vi "planarFFcircle.vi"(4 "ForceDesired":dbl, 6 "FM--FF":dbl[](array[numeric]), 7 "Radius":dbl, 8 "Center":dbl[](array[numeric]), 9 "ViconData":dbl[](array[numeric])) -> (2 "ActiveFF":bool, 3 "DesiredFM_FF":dbl[](array[numeric]))   [LabVIEW 2017]
uses:
  <vilib>/Analysis/_algsub.llb/Real Vector Norm.vi
  <vilib>/Analysis/NI_AALPro.lvlib
panel:
  out "Current_point":dbl[](array[numeric])
  out "center position":dbl[](array[numeric])
  # "Circle Force Field"
  # "INPUTS"
  # "OUTPUTS:"
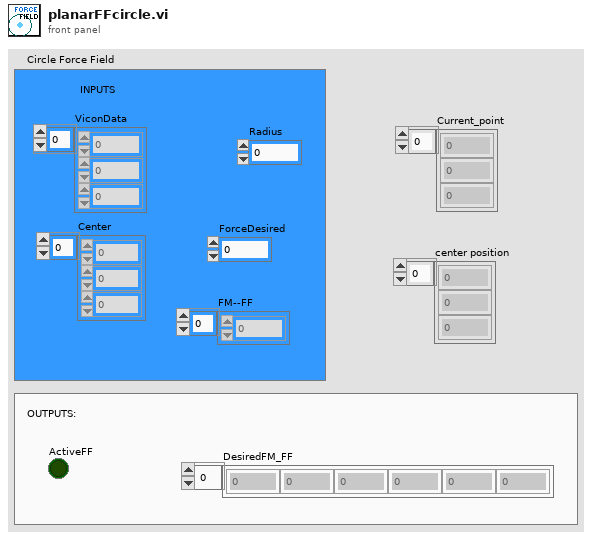
[diagram p1: front panel]
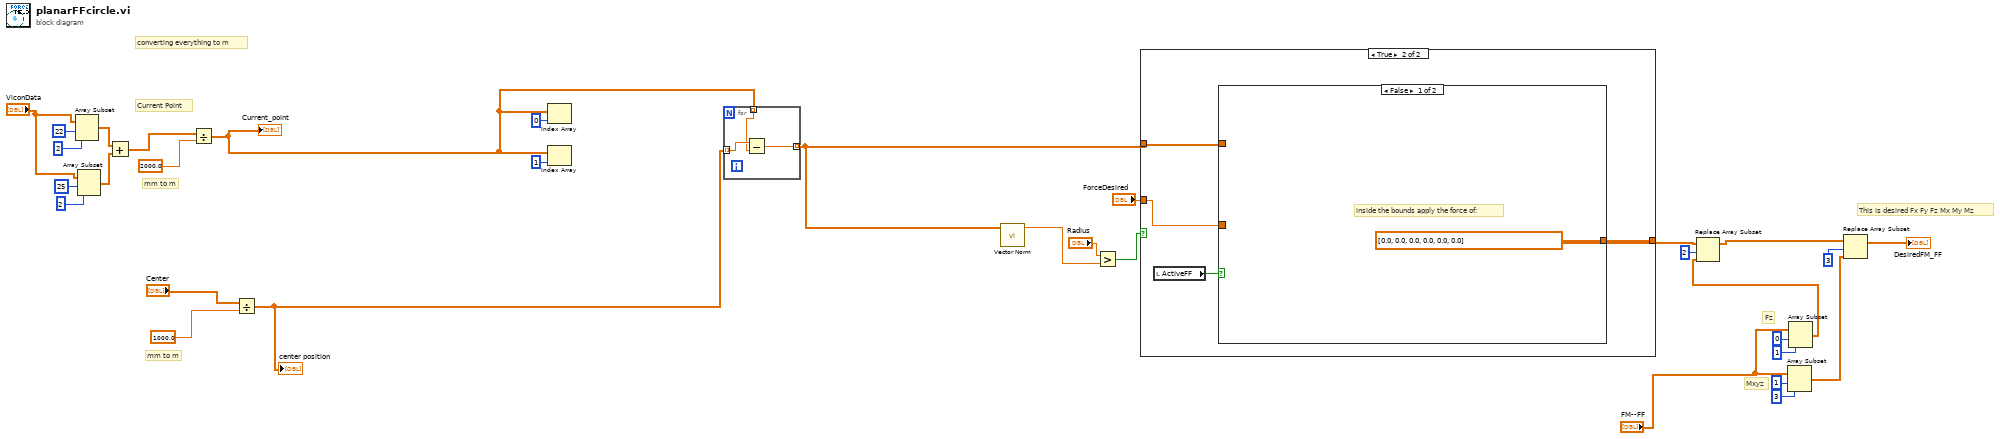
[diagram p0: block diagram]
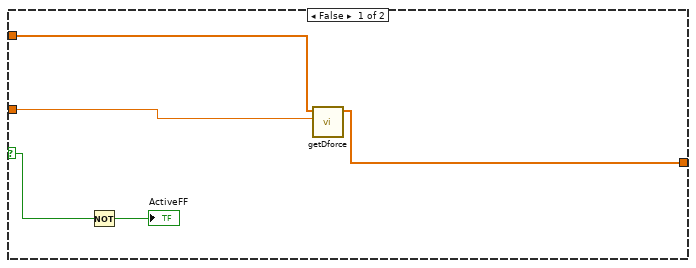
[diagram p2: hidden frame]
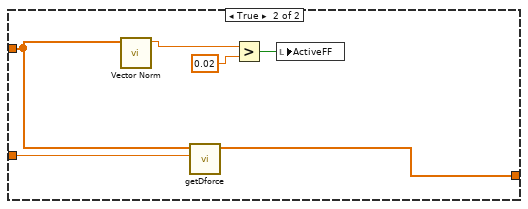
[diagram p3: hidden frame]
diagram:
  # "Current Point"
  # "mm to m"
  # "This is desired Fx Fy Fz Mx My Mz"
  # "converting everything to m"
  # "Fz"
  # "Mxyz"
  # "mm to m"
  n1 = Array Subset(array="ViconData", index=22, length=2) -> (w10:dbl[])
  n2 = Array Subset(array="ViconData", index=25, length=2) -> (w9:dbl[])
  n3 = Add(x=w10, y=w9) -> (x+y=w8:dbl[])
  n4 = Divide(x=w8, y=2000.0) -> (x/y=w7:dbl[])
  "Current_point" <- w7
  n5 = Divide(x="Center", y=1000.0) -> (x/y=w18:dbl[])
  "center position" <- w18
  n6 = Index Array(array=w7, index=0) -> ()  [unwired: 1 out]
  n7 = Index Array(array=w7, index=1) -> ()  [unwired: 1 out]
  n8 = for {
    tunnel: w18 -> [w34] mode=indexing
    tunnel: w7 -> [w33] mode=indexing
    tunnel: [w35] -> w5 mode=indexing
    n9 = Subtract(x=w34, y=w33) -> (x-y=w35:dbl)
  }
  n10 = call-poly <vilib>:"Vector Norm.vi"("Input Vector"=w5) -> ("norm"=w3:dbl)  [unwired: 9 in, 1 out]
  n11 = Greater?(x="Radius", y=w3) -> (0:w2:bool)
  n12 = case shown="True" w2 {
    selector: w2 -> [w36 _]
    tunnel: [w38 w44] -> w21
    tunnel: w5 -> [w40 w42]
    tunnel: "ForceDesired" -> [w39 w41]
    frame False {
      n13 = Not(x=w36) -> (.not. x?=→"ActiveFF":bool)
      n14 = call "getDforce.vi"("ForceDesired"=w39, "Desired Direction"=w40) -> ("FX FY Fz 0 0 0"=w38:dbl[])  [unwired: 5 in]
    }
    frame True {
      n15 = local read "ActiveFF"() -> (w43:bool)
      n16 = case shown="False" w43 {
        tunnel: [dbl[] [0.0, 0.0, 0.0, 0.0, 0.0, 0.0] w51] -> w44
        tunnel: w42 -> [_ w46]
        tunnel: w41 -> [_ w47]
        frame False {
          # "inside the bounds apply the force of:"
        }
        frame True {
          n17 = call-poly <vilib>:"Vector Norm.vi"("Input Vector"=w46) -> ("norm"=w50:dbl)  [unwired: 9 in, 1 out]
          n18 = call "getDforce.vi"("ForceDesired"=w47, "Desired Direction"=w46) -> ("FX FY Fz 0 0 0"=w51:dbl[])  [unwired: 5 in]
          n19 = Greater?(x=w50, y=0.02) -> (0:w48:bool)
          n20 = local write "ActiveFF"(w48) -> ()
        }
      }
    }
  }
  n21 = Array Subset(array="FM--FF", index=1, length=3) -> (w23:dbl[])
  n22 = Array Subset(array="FM--FF", index=0, length=1) -> (w22:dbl[])
  n23 = Replace Array Subset(array=w21, new element=w22, index=2) -> (w29:dbl[])
  n24 = Replace Array Subset(array=w29, new element=w23, index=3) -> (→"DesiredFM_FF":dbl[])
